vi "Duplicate Joystick Event.vi"(1 "Joystick Event 2":cluster{"Timestamp":u32, "Input":T1}, 2 "Joystick Event 1":cluster{"Timestamp":u32, "Input":T1}) -> (0 "Duplicate":bool)   [LabVIEW 2012]
uses:
  Joystick Event.ctl
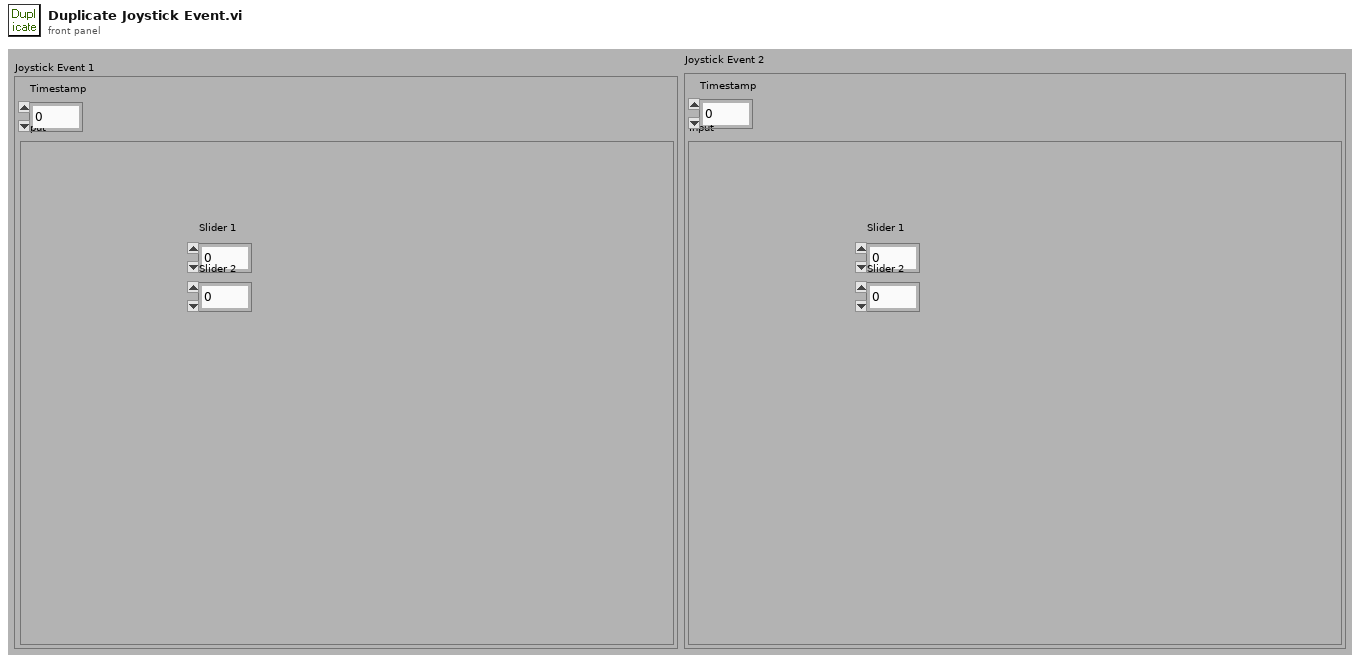
[diagram p1: front panel]
types:
  T1 = typedef "Joystick Event.ctl" = cluster{"Slider 1":dbl, "Slider 2":dbl}
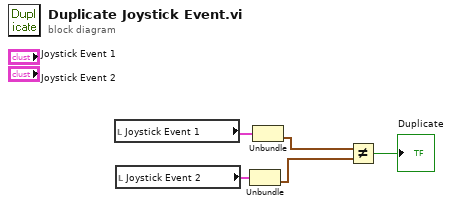
[diagram p0: block diagram]
diagram:
  n1 = local read "Joystick Event 1"() -> (w4:cluster{"Timestamp":u32, "Input":T1})
  n2 = local read "Joystick Event 2"() -> (w3:cluster{"Timestamp":u32, "Input":T1})
  n3 = Unbundle(w3) -> ("Input"=w2:T1)  [unwired: 1 out]
  n4 = Unbundle(w4) -> ("Input"=w1:T1)  [unwired: 1 out]
  n5 = Not Equal?(x=w1, y=w2) -> (x != y?=→"Duplicate":bool)
